vi "Configure Measurement Aperture.vi"(7 "Aperture Time (0.1s)":dbl=0.1, 8 "error in (no error)":errorcluster, 9 "Enable Aperture (F: Disable)":bool, 10 "Measurement Function (0: Continuity)":i32(ring) items=["Continuity", "Current AC", "Current DC", "Diode", "Frequency", "Resistance 4-wire", "Period", "Resistance 2-wire", "Temperature", "Voltage AC", "Voltage DC", "Voltage DC Ratio", "Capacitance"], 11 "VISA resource name":refnum<visa-resource-name>) -> (0 "error out":errorcluster, 3 "VISA resource name out":refnum<visa-resource-name>)   [LabVIEW 2013, in "Agilent 3446X Series.lvlib"]
doc: "Specifies the integration time in seconds (called aperture time) for dc current, resistance, fresistance, temperature, and dc voltage measurements.\n\n<b>Note: </b>\nAperture is only supported by the 34465A and 34470A .\nFor EDU34450A model, Only Frequency Aperture is supported."
uses:
  <instrlib>/Agilent 3446X Series/Agilent 3446X Series.lvlib
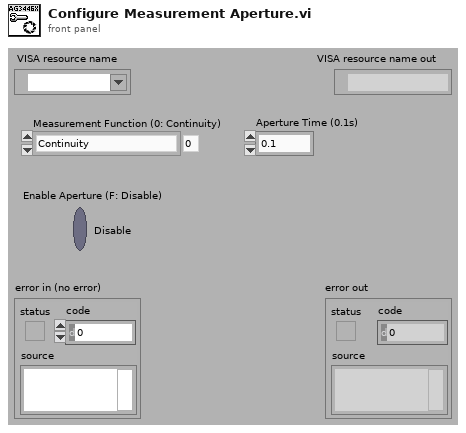
[diagram p1: front panel]
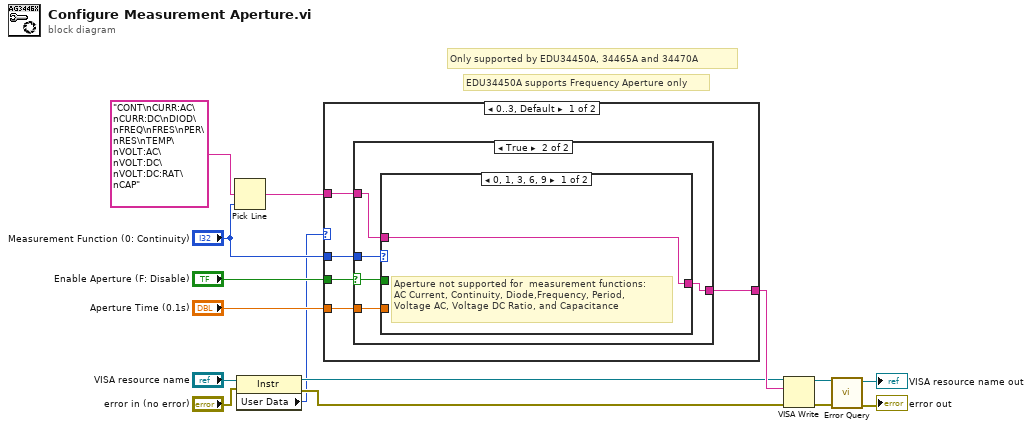
[diagram p0: block diagram]
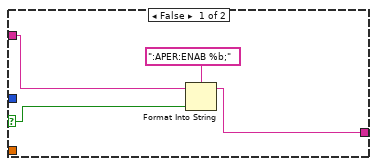
[diagram p2: hidden frame]
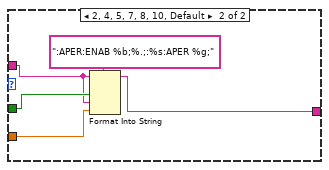
[diagram p3: hidden frame]
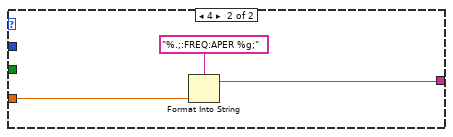
[diagram p4: hidden frame]
diagram:
  # "Only supported by EDU34450A, 34465A and 34470A"
  # "EDU34450A supports Frequency Aperture only"
  n1 = Pick Line(multi-line string="CONT\nCURR:AC\nCURR:DC\nDIOD\nFREQ\nFRES\nPER\nRES\nTEMP\nVOLT:AC\nVOLT:DC\nVOLT:DC:RAT\nCAP", line index="Measurement Function (0: Continuity)") -> (output string=w7:string)  [unwired: 1 out]
  n2 = property class="Instr"(reference="VISA resource name", error in="error in (no error)") -> (reference out=w3:refnum<visa-resource-name>, error out=w2:errorcluster, "User Data"=w1:u32)
  n3 = case shown="0..3, Default" w1 {
    tunnel: [w20 w36] -> w10
    tunnel: "Aperture Time (0.1s)" -> [w19 w37]
    tunnel: "Measurement Function (0: Continuity)" -> [w18 _]
    tunnel: w7 -> [w17 _]
    tunnel: "Enable Aperture (F: Disable)" -> [w16 _]
    frame 0..3, Default {
      n4 = case shown="True" w16 {
        selector: w16 -> [w21 w25]
        tunnel: [w22 w29] -> w20
        tunnel: w19 -> [_ w28]
        tunnel: w18 -> [_ w27]
        tunnel: w17 -> [w24 w26]
        frame False {
          n5 = Format Into String(format string=":APER:ENAB %b;", initial string=w24, w21) -> (resulting string=w22:string)  [unwired: 1 in, 1 out]
        }
        frame True {
          n6 = case shown="0, 1, 3, 6, 9" w27 {
            tunnel: [w30 w32] -> w29
            tunnel: w28 -> [_ w33]
            tunnel: w26 -> [w30 w31]
            tunnel: w25 -> [_ w34]
            frame 0, 1, 3, 6, 9 {
              # "Aperture not supported for  measurement functions:\nAC Current, Continuity, Diode,Frequency, Period, \nVoltage AC, Voltage DC Ratio, and Capacitance"
            }
            frame 2, 4, 5, 7, 8, 10, Default {
              n7 = Format Into String(format string=":APER:ENAB %b;%.;:%s:APER %g;", initial string=w31, w34, w31, w33) -> (resulting string=w32:string)  [unwired: 1 in, 1 out]
            }
          }
        }
      }
    }
    frame 4 {
      n8 = Format Into String(format string="%.;:FREQ:APER %g;", w37) -> (resulting string=w36:string)  [unwired: 2 in, 1 out]
    }
  }
  n9 = VISA Write(VISA resource name=w3, write buffer=w10, error in (no error)=w2) -> (VISA resource name out=w14:refnum<visa-resource-name>, error out=w13:errorcluster)  [unwired: 1 out]
  n10 = call <instrlib>:"Error Query.vi"("error in (no error)"=w13, "VISA resource name"=w14) -> ("error out"=→"error out":errorcluster, "VISA resource name out"=→"VISA resource name out":refnum<visa-resource-name>)  [unwired: 6 in, 2 out]
